vi "sensor fahren test.vi"() -> ()   [LabVIEW 2016]
uses:
  <vilib>/myRIO/Instrument Drivers/Onboard IO/PWM/typedefs/PWM Reference.ctl
  <vilib>/myRIO/Common/Instrument Driver Framework/Utilities/typedefs/myRIO Generic Hardware Reference.ctl
  <vilib>/myRIO/Common/Instrument Driver Framework/Utilities/typedefs/Hardware Version Enum.ctl
  <vilib>/myRIO/Common/Instrument Driver Framework/Utilities/typedefs/myRIO v1.0 Reference.ctl
  <vilib>/myRIO/Common/Instrument Driver Framework/Utilities/typedefs/Generic FPGA Reference.ctl
  <vilib>/myRIO/Common/Instrument Driver Framework/myRIO v1.0/PWM/typedefs/PWM Channels Enum.ctl
  <vilib>/myRIO/Instrument Drivers/Onboard IO/PWM/typedefs/PWM Configuration.ctl
  <vilib>/userdefined/High Color/nirio_resource_hc.ctl
  <vilib>/myRIO/Instrument Drivers/Onboard IO/AI/typedefs/AI Reference.ctl
  <vilib>/myRIO/Common/Instrument Driver Framework/myRIO v1.0/AI/typedefs/AI Channels List.ctl
  <vilib>/myRIO/Common/Instrument Driver Framework/myRIO v1.0/AI/typedefs/AI Channels Enum.ctl
  <vilib>/myRIO/Common/Instrument Driver Framework/Utilities/typedefs/Analog Scaling Constants List.ctl
  <vilib>/myRIO/Common/Instrument Driver Framework/Utilities/typedefs/Analog Scaling Constants.ctl
  <vilib>/myRIO/Common/Instrument Driver Framework/myRIO v1.0/PWM/vis/myRIO v1.1 Open PWM.vi
  <vilib>/myRIO/Common/Instrument Driver Framework/Utilities/vis/Is FPGA Ref Available.vi
  <vilib>/myRIO/Common/Instrument Driver Framework/myRIO v1.0/AI/vis/myRIO v1.1 Open AI.vi
  <vilib>/myRIO/Instrument Drivers/Onboard IO/AI/vis/Read.vi
  <vilib>/myRIO/Common/Instrument Driver Framework/Utilities/vis/Validate Channels.vi
  <vilib>/myRIO/Common/Instrument Driver Framework/myRIO v1.0/PWM/vis/myRIO v1.0 Reserve PWM.vi
  <vilib>/myRIO/Common/Instrument Driver Framework/myRIO v1.0/AI/vis/myRIO v1.0 Reserve AI.vi
  <vilib>/myRIO/Common/Instrument Driver Framework/myRIO v1.0/PWM/vis/myRIO v1.0 Build MUX Configuration PWM.vi
  <vilib>/myRIO/Common/Instrument Driver Framework/myRIO v1.0/Resource Manager/vis/myRIO v1.0 Reserve Channel List.vi
  <vilib>/myRIO/Common/Instrument Driver Framework/myRIO v1.0/AI/vis/myRIO v1.0 Build MUX Configuration AI.vi
  <vilib>/myRIO/Common/Instrument Driver Framework/myRIO v1.0/Resource Manager/vis/myRIO v1.0 Create Configuration List.vi
  <vilib>/myRIO/Common/Instrument Driver Framework/myRIO v1.0/Resource Manager/vis/myRIO v1.0 Reserve Channel.vi
  <vilib>/myRIO/Common/Instrument Driver Framework/myRIO v1.0/Resource Manager/vis/myRIO v1.0 Unreserve Channel.vi
  <vilib>/myRIO/Common/Instrument Driver Framework/myRIO v1.0/Resource Manager/vis/myRIO v1.0 Build Mutex Name.vi
  <vilib>/Utility/VariantDataType/GetNumericInfo.vi
  <vilib>/Utility/error.llb/Error Cluster From Error Code.vi
  <vilib>/myRIO/Common/Instrument Driver Framework/myRIO v1.0/myRIO v1.1 Open.vi
  <vilib>/myRIO/Common/Instrument Driver Framework/Utilities/vis/IO Manager.vi
  <vilib>/myRIO/Common/Instrument Driver Framework/Utilities/vis/Configuration Manager.vi
  <vilib>/myRIO/Common/Instrument Driver Framework/myRIO v1.0/Resource Manager/vis/myRIO v1.0 Configure IO.vi
  <vilib>/myRIO/Common/Instrument Driver Framework/myRIO v1.0/myRIO v1.0 Close.vi
  <vilib>/myRIO/Common/Instrument Driver Framework/myRIO v1.0/AI/vis/myRIO v1.0 Get Scaling Constants AI.vi
  <vilib>/myRIO/Common/Instrument Driver Framework/myRIO v1.0/AI/vis/myRIO v1.0 Read AI.vi
  <vilib>/myRIO/Common/Instrument Driver Framework/myRIO v1.0/PWM/vis/myRIO v1.0 Write PWM.vi
  <vilib>/myRIO/Instrument Drivers/Onboard IO/PWM/vis/myRIO PWM Open.xnode
  <vilib>/myRIO/Express VI/Onboard IO/AI/AI Express VI.xnode
  <vilib>/myRIO/Instrument Drivers/Onboard IO/AI/vis/myRIO AI Open.xnode
  <vilib>/myRIO/Instrument Drivers/Onboard IO/PWM/PWM.lvlib
  <vilib>/myRIO/Instrument Drivers/Onboard IO/AI/AI.lvlib
panel:
  out "B/AI1 (Pin 5) 2":dbl(graph)
  out "B/AI1 (Pin 5)":dbl
  out "Distanz":dbl
  in  "Knob":dbl(knob)=0.3 scale=0.0..0.5
  in  "stop":bool
  in  "Frequenz Motor":dbl=200.0
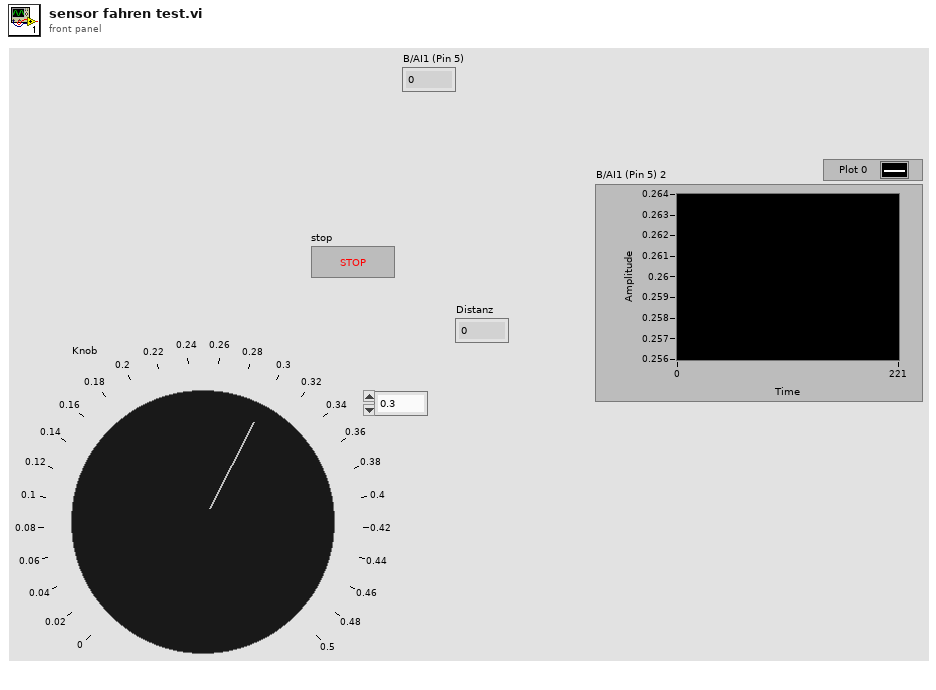
[diagram p1: front panel]
types:
  T1 = typedef "PWM.lvlib/PWM Reference.ctl" = cluster{"myRIO Reference":T2, "PWM Channels Enum":T6, "PWM Configuration":T7}
  T2 = typedef "myRIO Generic Hardware Reference.ctl" = cluster{"myRIO Model":T3, "myRIO Hardware Reference":T4}
  T3 = typedef "Hardware Version Enum.ctl" = enum16{"Unknown", "myRIO-1900", "myRIO-1950", "roboRIO", "NI ELVIS RIO CM"}
  T4 = typedef "myRIO v1.0 Reference.ctl" = cluster{"Generic FPGA Reference":T5, "Allow multiple opens":bool}
  T5 = typedef "Generic FPGA Reference.ctl" = refnum<k20>
  T6 = typedef "PWM Channels Enum.ctl" = enum16{"Not Connected", "C/PWM0", "C/PWM1", "A/PWM0", "A/PWM1", "A/PWM2", "B/PWM0", "B/PWM1", "B/PWM2", "PWM/PWM0", "PWM/PWM1", "PWM/PWM2", "PWM/PWM3", "PWM/PWM4", "PWM/PWM5", "PWM/PWM6", "PWM/PWM7", "PWM/PWM8", "PWM/PWM9"}
  T7 = typedef "PWM.lvlib/PWM Configuration.ctl" = cluster{"Frequency":dbl, "Duty Cycle":dbl}
  T8 = typedef "AI.lvlib/AI Reference.ctl" = cluster{"myRIO Reference":T2, "AI Channels List":T9, "AI Scaling Constants List":T11}
  T9 = typedef "AI Channels List.ctl" = T10[]
  T10 = typedef "AI Channels Enum.ctl" = enum16{"Not Connected", "AudioIn/Left", "AudioIn/Right", "C/AI0", "C/AI1", "A/AI0", "A/AI1", "A/AI2", "A/AI3", "B/AI0", "B/AI1", "B/AI2", "B/AI3", "AI/AI0", "AI/AI1", "AI/AI2", "AI/AI3"}
  T11 = typedef "Analog Scaling Constants List.ctl" = T12[]
  T12 = typedef "Analog Scaling Constants.ctl" = cluster{"LSB Weight (Volts)":dbl, "Offset (Volts)":dbl, "Signed?":bool}
  T13 = typedef "nirio_resource_hc.ctl" = tag
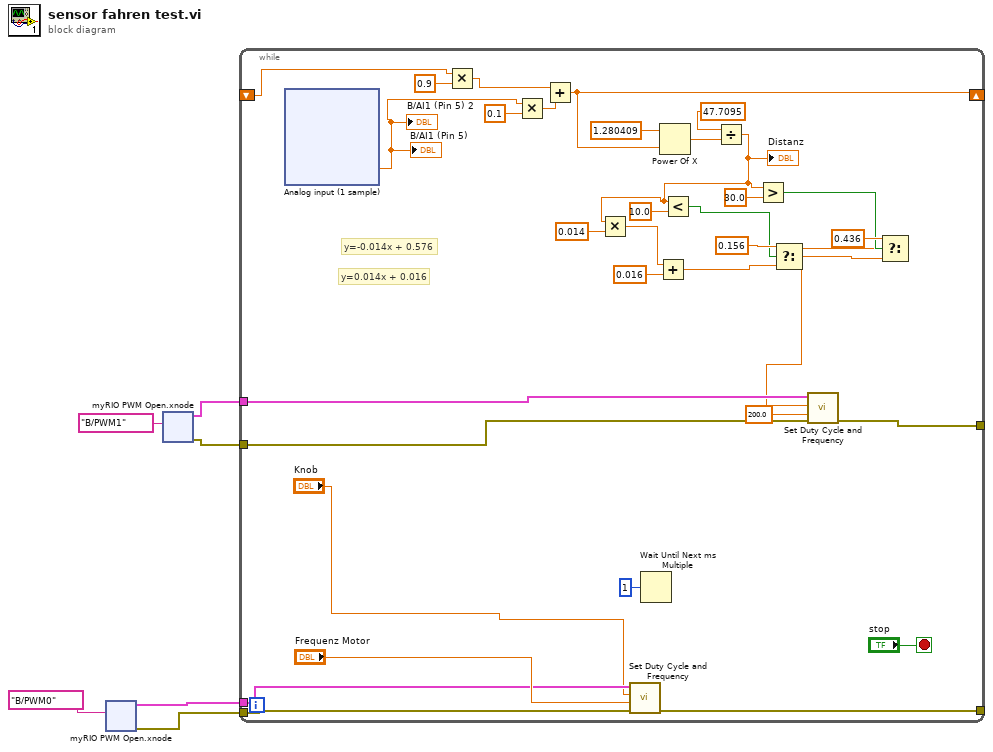
[diagram p0: block diagram]
diagram:
  n1 = xnode "myRIO PWM Open.xnode"("Channel Name"=tag "B/PWM0") -> ("error out"=w4:errorcluster, "PWM Ref Out"=w5:T1)  [unwired: 2 in]
  n2 = xnode "myRIO PWM Open.xnode"("Channel Name"=tag "B/PWM1") -> ("error out"=w1:errorcluster, "PWM Ref Out"=w2:T1)  [unwired: 2 in]
  n3 = while {
    tunnel: [w40] -> _
    tunnel: w5 -> [w37]
    tunnel: w4 -> [w36]
    shift-right: [w27] -> _
    shift-left: _ -> [w29]
    tunnel: w2 -> [w25]
    tunnel: w1 -> [w24]
    tunnel: [w23] -> _
    stop <- "stop" stop-if-true
    # "y=0.014x + 0.016"
    # "y=-0.014x + 0.576"
    n4 = xnode "Analog input (1 sample)"() -> ("B/AI1 (Pin 5)"=w7:dbl)  [unwired: 1 in, 1 out]
    "B/AI1 (Pin 5)" <- w7
    "B/AI1 (Pin 5) 2" <- w7
    n5 = Multiply(x=w29, y=0.9) -> (x*y=w31:dbl)
    n6 = Multiply(x=w7, y=0.1) -> (x*y=w30:dbl)
    n7 = Add(x=w31, y=w30) -> (x+y=w27:dbl)
    n8 = call <vilib>:"Set Duty Cycle and Frequency.vi"("error in (no error)"=w36, "Frequency [Hz]"="Frequenz Motor", "Duty Cycle"="Knob", "PWM Ref In"=w37) -> ("error out"=w40:errorcluster)  [unwired: 5 in, 1 out]
    n9 = Wait Until Next ms Multiple(millisecond multiple=u32 1 ("milliseconds to wait")) -> ()  [unwired: 1 out]
    n10 = Power Of X(1:w27, 2:1.280409 ("y")) -> (0:w33:dbl)
    n11 = Divide(x=47.7095, y=w33) -> (x/y=w11:dbl)
    "Distanz" <- w11
    n12 = Multiply(x=w11, y=0.014) -> (x*y=w21:dbl)
    n13 = Add(x=w21, y=0.016) -> (x+y=w19:dbl)
    n14 = Less?(x=w11, y=10.0) -> (x < y?=w14:bool)
    n15 = Greater?(x=w11, y=30.0) -> (0:w12:bool)
    n16 = Select(t=0.156, s=w14, f=w19) -> (s? t:f=w17:dbl)
    n17 = Select(t=0.436, s=w12, f=w17) -> (s? t:f=w10:dbl)
    n18 = call <vilib>:"Set Duty Cycle and Frequency.vi"("error in (no error)"=w24, "Frequency [Hz]"=200.0 ("y"), "Duty Cycle"=w10, "PWM Ref In"=w25) -> ("error out"=w23:errorcluster)  [unwired: 5 in, 1 out]
  }
